vi "Startup.vi"(6 "LabVIEW Web Service":refnum<class "Web Service.lvclass">) -> ()   [LabVIEW 2016]
uses:
  <vilib>/wsapi/Web Service.lvclass
  Classes/Request/Request.lvclass/Request.ctl
  Classes/Request/Read method.vi
  Classes/Request/Read params.vi
  Classes/Server/Add Response (Method Not Found from Request).vi
  Classes/Server/Add Response (Server Error from Request).vi
  Classes/params/params.lvclass
  Classes/Server/JSONRPC Server.lvclass
  Classes/Request/Request.lvclass
panel:
  out "error out":errorcluster
  # "Use the web service input terminal to call the VIs on the Service subpalette of the Web Services palette. Do not remove it from the connector pane unless you don't need access to the palette."
  # "Any additional terminals added to the connector pane of a startup VI will be ignored."
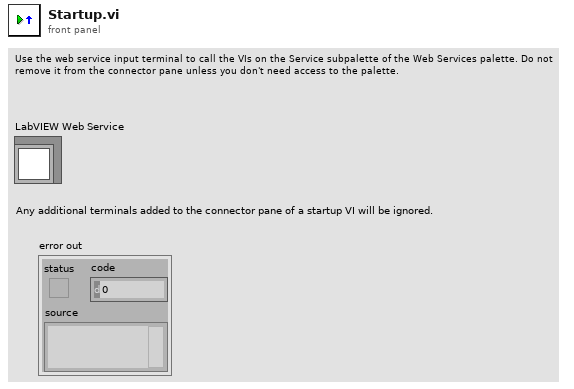
[diagram p1: front panel]
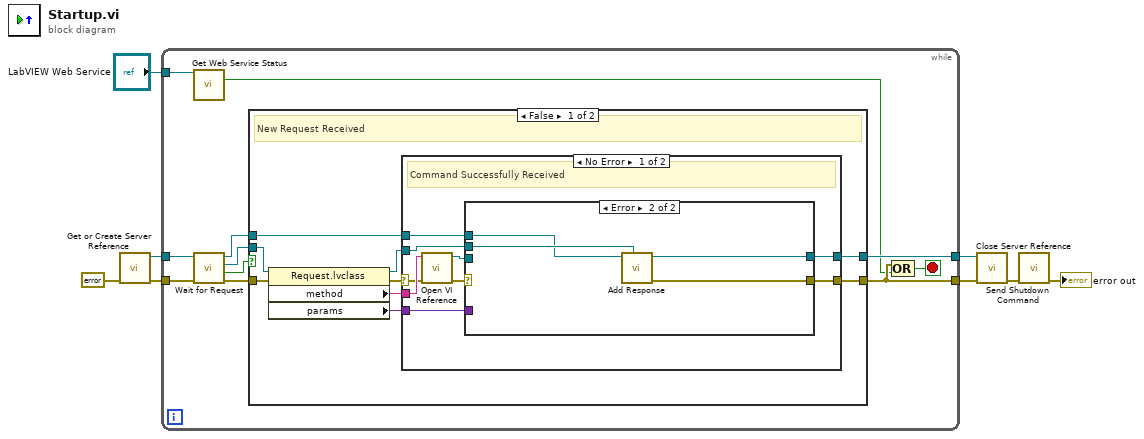
[diagram p0: block diagram]
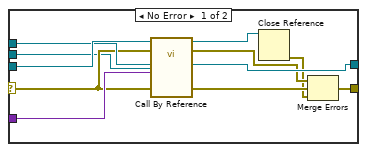
[diagram p2: hidden frame]
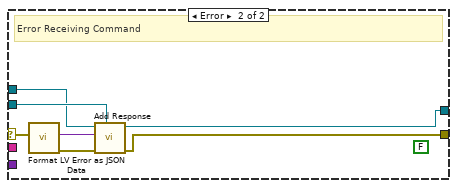
[diagram p3: hidden frame]
diagram:
  n1 = call "Get or Create Server Reference.vi"("error in (no error)"=errorcluster {"status"=FALSE, "code"=0, "source"=""} ("error constant")) -> ("error out"=w5:errorcluster, "Server Out"=w4:refnum<class "JSONRPC Server.lvclass">)  [unwired: 9 in]
  n2 = while {
    tunnel: w4 -> [w19]
    tunnel: w5 -> [w15]
    tunnel: [w12] -> w7
    tunnel: [w13] -> w6
    tunnel: "LabVIEW Web Service" -> [w9]
    stop <- w11 stop-if-true
    n3 = call <vilib>:"Get Web Service Status.vi"("LabVIEW Web Service"=w9) -> ("service stopping?"=w10:bool)  [unwired: 12 in, 2 out]
    n4 = call "Wait for Request.vi"("error in (no error)"=w15, "Server in"=w19) -> ("error out"=w14:errorcluster, "timed out?"=w16:bool, "Request"=w17:refnum<class "Request.lvclass">, "Server out"=w18:refnum<class "JSONRPC Server.lvclass">)  [unwired: 6 in]
    n5 = case shown="False" w16 {
      tunnel: w18 -> [w22 w60]
      tunnel: w17 -> [w28 _]
      tunnel: w14 -> [w25 w61]
      tunnel: [w23 w61] -> w12
      tunnel: [w21 w60] -> w13
      frame False {
        # "New Request Received"
        n6 = property class="Request.lvclass"(reference=w28, error in=w25) -> (reference out=w20:refnum<class "Request.lvclass">, error out=w24:errorcluster, "method"=w27:string, "params"=w26:variant)
        n7 = case shown="No Error" w24 {
          selector: w24 -> [w32 w54]
          tunnel: w27 -> [w37 _]
          tunnel: w26 -> [w34 _]
          tunnel: [w30 w56] -> w23
          tunnel: w22 -> [w35 w58]
          tunnel: [w33 w57] -> w21
          tunnel: w20 -> [w29 w59]
          frame No Error {
            # "Command Successfully Received"
            n8 = call "Open VI Reference.vi"("error in (no error)"=w32, "method"=w37) -> ("error out"=w31:errorcluster, "VI out"=w36:refnum<vi>)  [unwired: 8 in]
            n9 = case shown="Error" w31 {
              selector: w31 -> [w44 _]
              tunnel: w36 -> [w48 _]
              tunnel: w35 -> [w47 w51]
              tunnel: w34 -> [w46 _]
              tunnel: [w45 w50] -> w33
              tunnel: [w41 w49] -> w30
              tunnel: w29 -> [w40 w52]
              frame No Error {
                n10 = call-by-ref "?"(reference=w48, error in=w44, "Request in"=w40, 8:"error in (no error)"=w44, "params"=w46, "Server in"=w47) -> (reference out=w39:refnum<vi>, error out=w43:errorcluster, 0:"error out"=w42:errorcluster, "JSONRPC Server out"=w45:refnum<class "JSONRPC Server.lvclass">)  [unwired: 6 in]
                n11 = Close Reference(reference=w39) -> (error out=w38:errorcluster)  [unwired: 1 in]
                n12 = Merge Errors(w43, w42, w38) -> (w41:errorcluster)
              }
              frame Error {
                n13 = call-poly "Add Response.vi"("Request"=w52, "Server in"=w51) -> ("error out"=w49:errorcluster, "Server out"=w50:refnum<class "JSONRPC Server.lvclass">)  [unwired: 7 in, 1 out]
              }
            }
          }
          frame Error {
            (unwired) FALSE
            # "Error Receiving Command"
            n14 = call "Format LV Error as JSON Data.vi"("error in"=w54) -> ("error out"=w55:errorcluster, "Error Data Out"=w53:variant)  [unwired: 9 in]
            n15 = call-poly "Add Response.vi"("Request"=w59, "error in (no error)"=w55, "data"=w53, "Server in"=w58) -> ("error out"=w56:errorcluster, "Server out"=w57:refnum<class "JSONRPC Server.lvclass">)  [unwired: 5 in, 1 out]
          }
        }
      }
      frame True {
        # "Timeout while waiting for new Requests"
      }
    }
    n16 = Compound Arithmetic op=OR(w12, w10) -> (w11:bool)
  }
  n17 = call-dynamic "Close Server Reference.vi"("error in (no error)"=w7, "Server in"=w6) -> ("error out"=w3:errorcluster)  [unwired: 9 in]
  n18 = call "Send Shutdown Command.vi"("error in (no error)"=w3) -> ("error out"=→"error out":errorcluster)  [unwired: 10 in]
